vi "Classify Goal Side 624 Aerial Assist.vi"(4 "Left Cam?":bool, 7 "Vision Mode":T1 caption="Vision Mode (Reported by Robot)", 10 "Targets in":T3(array[cluster])) -> (2 "Targets out":T3(array[cluster]))   [LabVIEW 2013]
uses:
  TargetType.ctl
  Common Code/Vision Mode.ctl
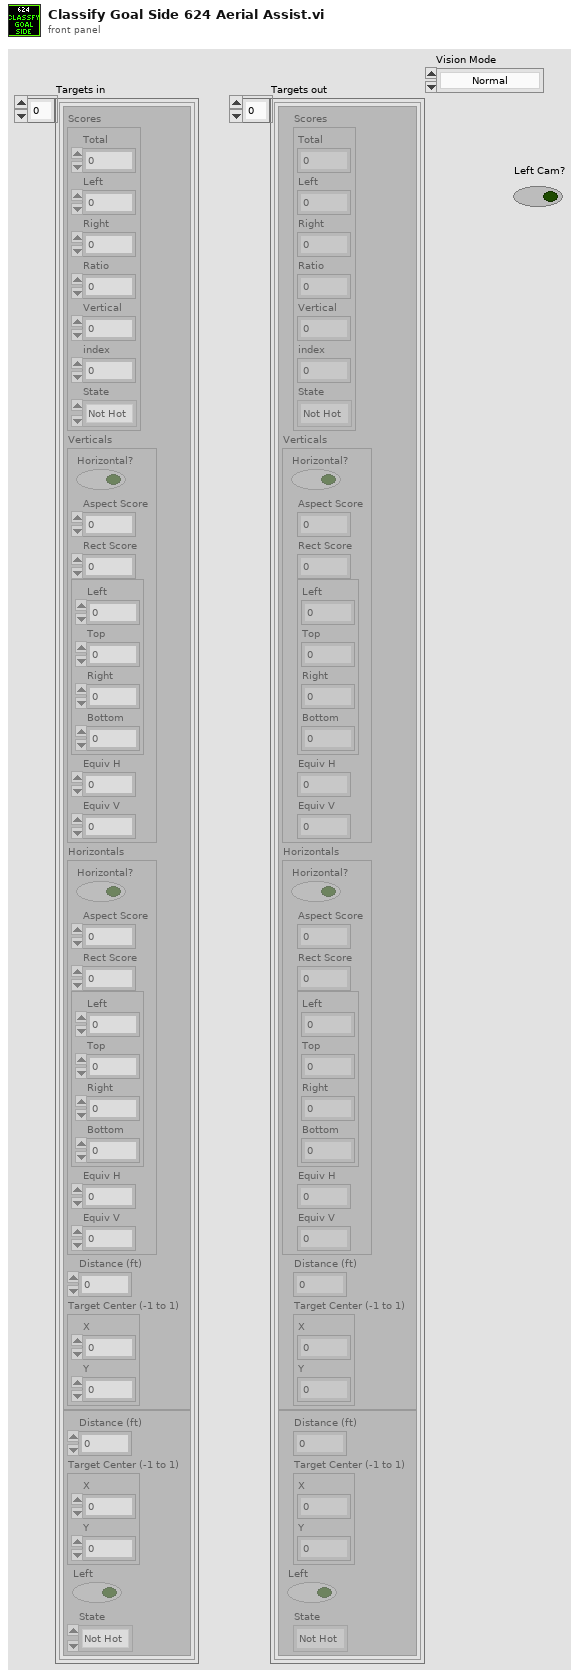
[diagram p1: front panel]
types:
  T1 = typedef "Vision Mode.ctl" = enum16{"Normal", "Extreme Left", "Extreme Right"}
  T2 = typedef "TargetType.ctl" = enum16{"Not Hot", "Hot"}
  T3 = cluster{cluster{"Scores":cluster{"Total":dbl, "Left":dbl, "Right":dbl, "Ratio":dbl, "Vertical":dbl, "index":i32, "State":T2}, "Verticals":cluster{"Horizontal?":bool, "Aspect Score":dbl, "Rect Score":dbl, cluster{"Left":dbl, "Top":dbl, "Right":dbl, "Bottom":dbl}, "Equiv H":dbl, "Equiv V":dbl}, "Horizontals":cluster{"Horizontal?":bool, "Aspect Score":dbl, "Rect Score":dbl, cluster{"Left":dbl, "Top":dbl, "Right":dbl, "Bottom":dbl}, "Equiv H":dbl, "Equiv V":dbl}, "Distance (ft)":dbl, "Target Center (-1 to 1)":cluster{"X":dbl, "Y":dbl}}, cluster{"Distance (ft)":dbl, "Target Center (-1 to 1)":cluster{"X":dbl, "Y":dbl}, "Left":bool, "State":T2}}[]
  T4 = cluster{"Distance (ft)":dbl, "Target Center (-1 to 1)":cluster{"X":dbl, "Y":dbl}, "Left":bool, "State":T2}
  T5 = cluster{"Scores":cluster{"Total":dbl, "Left":dbl, "Right":dbl, "Ratio":dbl, "Vertical":dbl, "index":i32, "State":T2}, "Verticals":cluster{"Horizontal?":bool, "Aspect Score":dbl, "Rect Score":dbl, cluster{"Left":dbl, "Top":dbl, "Right":dbl, "Bottom":dbl}, "Equiv H":dbl, "Equiv V":dbl}, "Horizontals":cluster{"Horizontal?":bool, "Aspect Score":dbl, "Rect Score":dbl, cluster{"Left":dbl, "Top":dbl, "Right":dbl, "Bottom":dbl}, "Equiv H":dbl, "Equiv V":dbl}, "Distance (ft)":dbl, "Target Center (-1 to 1)":cluster{"X":dbl, "Y":dbl}}
  T6 = cluster{cluster{"Scores":cluster{"Total":dbl, "Left":dbl, "Right":dbl, "Ratio":dbl, "Vertical":dbl, "index":i32, "State":T2}, "Verticals":cluster{"Horizontal?":bool, "Aspect Score":dbl, "Rect Score":dbl, cluster{"Left":dbl, "Top":dbl, "Right":dbl, "Bottom":dbl}, "Equiv H":dbl, "Equiv V":dbl}, "Horizontals":cluster{"Horizontal?":bool, "Aspect Score":dbl, "Rect Score":dbl, cluster{"Left":dbl, "Top":dbl, "Right":dbl, "Bottom":dbl}, "Equiv H":dbl, "Equiv V":dbl}, "Distance (ft)":dbl, "Target Center (-1 to 1)":cluster{"X":dbl, "Y":dbl}}, cluster{"Distance (ft)":dbl, "Target Center (-1 to 1)":cluster{"X":dbl, "Y":dbl}, "Left":bool, "State":T2}}
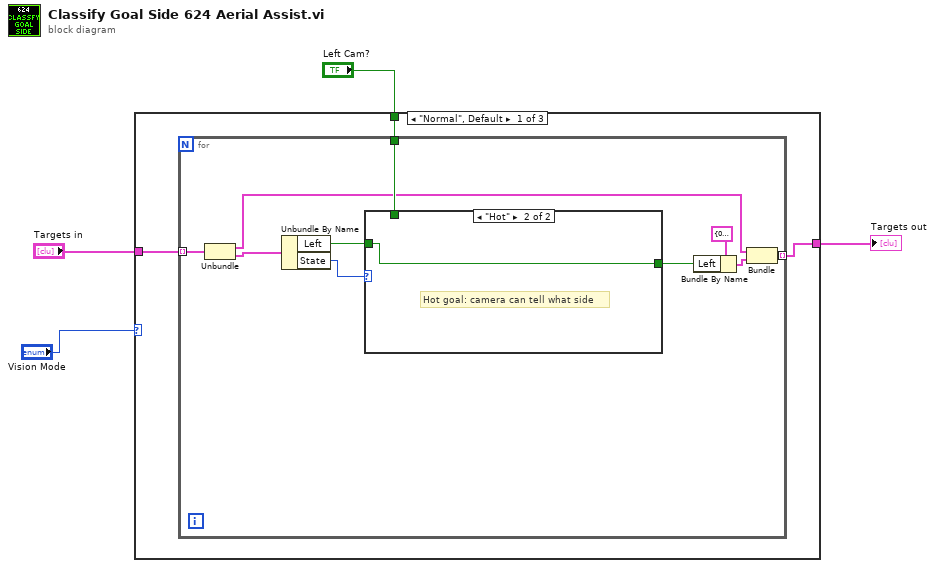
[diagram p0: block diagram]
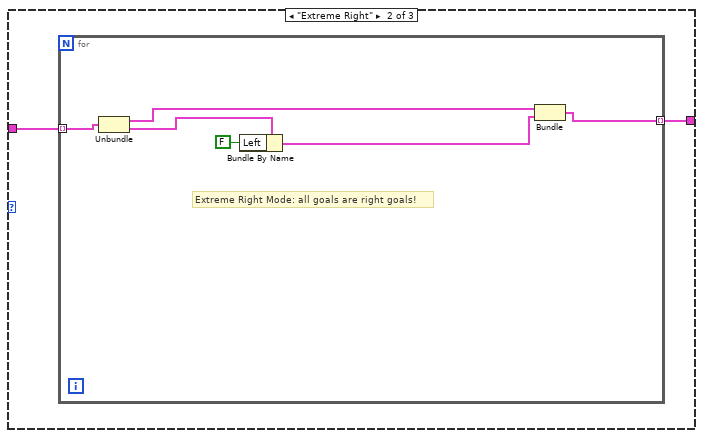
[diagram p3: hidden frame]
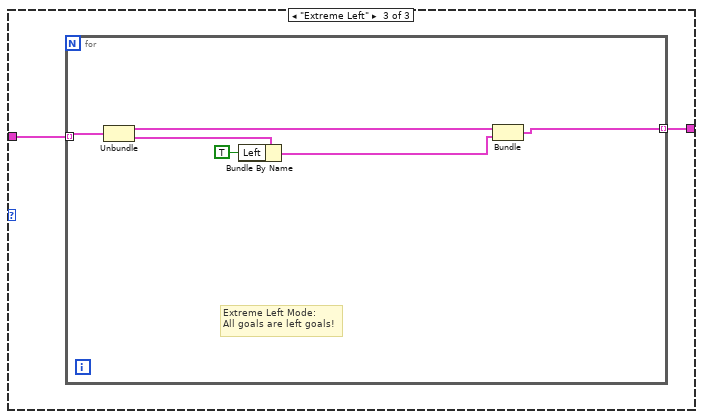
[diagram p4: hidden frame]
diagram:
  n1 = case shown="\"Normal\", Default" "Vision Mode" {
    tunnel: "Targets in" -> [w7 w21 w29]
    tunnel: "Left Cam?" -> [w6 _ _]
    tunnel: [w5 w20 w28] -> w1
    frame "Normal", Default {
      n2 = for {
        tunnel: w7 -> [w17] mode=indexing
        tunnel: w6 -> [w11]
        tunnel: [w8] -> w5 mode=indexing
        n3 = Unbundle(w17) -> (w9:T5, w14:T4)
        n4 = Unbundle By Name(w14) -> ("Left"=w15:bool, "State"=w16:T2)
        n5 = case shown="\"Hot\"" w16 {
          tunnel: w15 -> [_ w19]
          tunnel: [w18 w19] -> w12
          tunnel: w11 -> [w18 _]
          frame "Not Hot", Default {
            # "Not hot: make educated guess by which\ncam the goal appears in"
          }
          frame "Hot" {
            # "Hot goal: camera can tell what side"
          }
        }
        n6 = Bundle By Name(cluster=T4 {"Distance (ft)"=0.0, "Target Center (-1 to 1)"={"X"=0.0, "Y"=0.0}, "Left"=FALSE, "State"=enum."Not Hot"}, "Left"=w12) -> (w10:T4)
        n7 = Bundle(w9, w10) -> (w8:T6)  [unwired: 1 in]
      }
    }
    frame "Extreme Right" {
      n8 = for {
        tunnel: w21 -> [w27] mode=indexing
        tunnel: [w22] -> w20 mode=indexing
        # "Extreme Right Mode: all goals are right goals!"
        n9 = Unbundle(w27) -> (w24:T5, w26:T4)
        n10 = Bundle By Name(cluster=w26, "Left"=FALSE) -> (w23:T4)
        n11 = Bundle(w24, w23) -> (w22:T6)  [unwired: 1 in]
      }
    }
    frame "Extreme Left" {
      n12 = for {
        tunnel: w29 -> [w35] mode=indexing
        tunnel: [w30] -> w28 mode=indexing
        # "Extreme Left Mode:\nAll goals are left goals!"
        n13 = Unbundle(w35) -> (w31:T5, w34:T4)
        n14 = Bundle By Name(cluster=w34, "Left"=TRUE) -> (w32:T4)
        n15 = Bundle(w31, w32) -> (w30:T6)  [unwired: 1 in]
      }
    }
  }
  "Targets out" <- w1
